vi "EmptyMenu.vi"(8 "error in (no error)":errorcluster, 11 "MGI_TrayIcon in":refnum<class "MGI_TrayIcon.lvclass">) -> (0 "error out":errorcluster, 3 "MGI_TrayIcon out":refnum<class "MGI_TrayIcon.lvclass">)   [LabVIEW 2016, in "MGI_TrayIcon.lvclass"]
doc: "Authored by Derek E. Trepanier\nsupport@mooregoodideas.com\nwww.mooregoodideas.com\n\nCopyright (c) 2012, Moore Good Ideas, Inc.\n\nAll rights reserved.\n\nRedistribution and use in source and binary forms, with or without modification, are permitted provided that the following conditions are met:\n\n * Redistributions of source code must retain the above copyright notice, this list of conditions and the following disclaimer.\n * Redistributions in binary form must reproduce the above copyright notice, this list of conditions and the following disclaimer in the documentation and/or other materials provided with the distribution.\n * Neither the name of Moore Good Ideas, Inc. nor the names of its contributors may be used to endorse or promote products derived from this software without specific prior written permission.\n\nTHIS SOFTWARE IS PROVIDED BY THE COPYRIGHT HOLDERS AND CONTRIBUTORS \"AS IS\" AND ANY EXPRESS OR IMPLIED WARRANTIES, INCLUDING, BUT NOT LIMITED TO, THE IMPLIED WARRANTIES OF MERCHANTABILITY AND FITNESS FOR A PARTICULAR PURPOSE ARE DISCLAIMED. IN NO EVENT SHALL THE COPYRIGHT OWNER OR CONTRIBUTORS BE LIABLE FOR ANY DIRECT, INDIRECT, INCIDENTAL, SPECIAL, EXEMPLARY, OR CONSEQUENTIAL DAMAGES (INCLUDING, BUT NOT LIMITED TO, PROCUREMENT OF SUBSTITUTE GOODS OR SERVICES; LOSS OF USE, DATA, OR PROFITS; OR BUSINESS INTERRUPTION) HOWEVER CAUSED AND ON ANY THEORY OF LIABILITY, WHETHER IN CONTRACT, STRICT LIABILITY, OR TORT (INCLUDING NEGLIGENCE OR OTHERWISE) ARISING IN ANY WAY OUT OF THE USE OF THIS SOFTWARE, EVEN IF ADVISED OF THE POSSIBILITY OF SUCH DAMAGE."
uses:
  <userlib>/_MGI/Menu Building/MenuTypes/TrayIcon/MGI_TrayIcon.lvclass
  System.Windows.Forms
  <userlib>/_MGI/Menu Building/MenuTypes/TrayIcon/MGI_TrayIcon.lvclass/MGI_TrayIcon.ctl
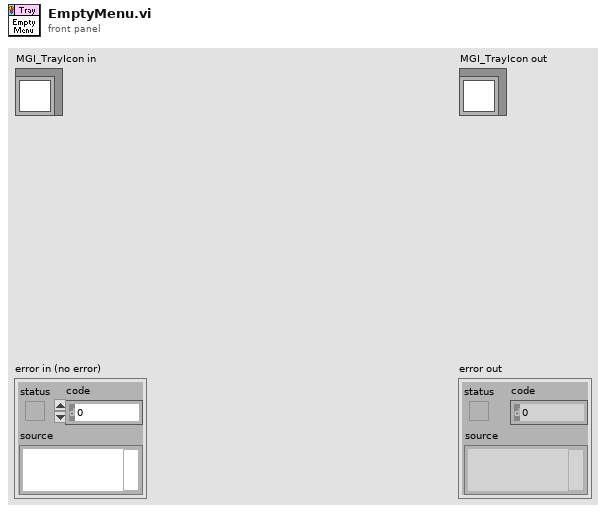
[diagram p1: front panel]
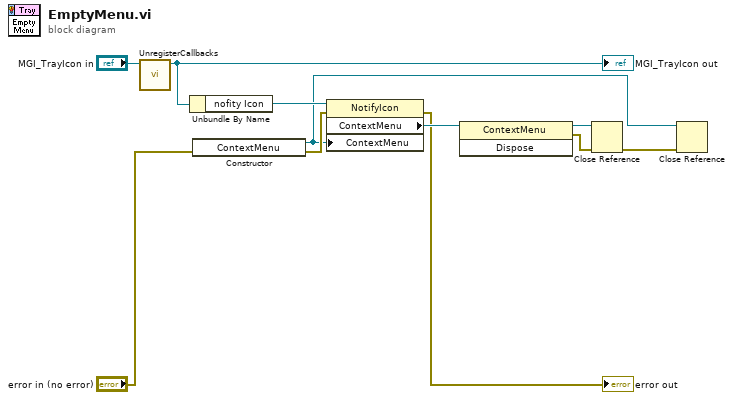
[diagram p0: block diagram]
diagram:
  n1 = call <userlib>:"UnregisterCallbacks.vi"("MGI_TrayIcon in"="MGI_TrayIcon in") -> ("MGI_TrayIcon out"=w3:refnum<class "MGI_TrayIcon.lvclass">)  [unwired: 9 in, 1 out]
  "MGI_TrayIcon out" <- w3
  n2 = Unbundle By Name(w3) -> ("nofity Icon"=w11:refnum<k24>)
  n3 = constructor class="ContextMenu"(error in="error in (no error)") -> (reference out=w1:refnum<k24>, error out=w6:errorcluster)  [unwired: 2 in, 1 out]
  n4 = property class="NotifyIcon"(reference=w11, error in=w6, "ContextMenu"=w1) -> (error out=→"error out":errorcluster, "ContextMenu"=w10:refnum<k24>)  [unwired: 1 out]
  n5 = invoke class="ContextMenu" method="Dispose"(reference=w10) -> (reference out=w9:refnum<k24>, error out=w8:errorcluster)  [unwired: 2 in, 1 out]
  n6 = Close Reference(reference=w9, error in (no error)=w8) -> (error out=w2:errorcluster)
  n7 = Close Reference(reference=w1, error in (no error)=w2) -> ()  [unwired: 1 out]
